vi "LOGIC_CheckStopCond.vi"(8 "error in (no error)":errorcluster, 11 "Database RefNum in":T1) -> (0 "error out":errorcluster)   [LabVIEW 2016]
uses:
  DBSHAND/private/vis/DatabaseHand_RefNum.ctl
  DBSHAND/private/vis/DatabaseHand_Element_Get(bool).vi
  DBSHAND/private/vis/DatabaseHand_Element_Set(I32).vi
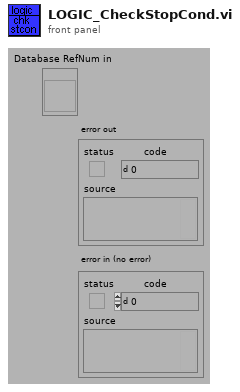
[diagram p1: front panel]
types:
  T1 = typedef "DatabaseHand_RefNum.ctl" = refnum<vi>
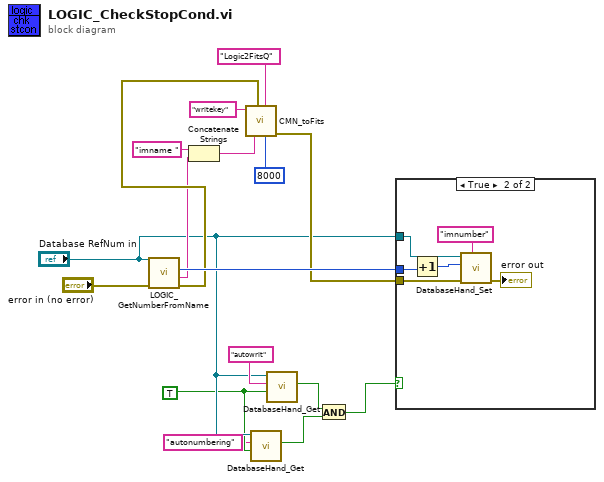
[diagram p0: block diagram]
diagram:
  w4 = TRUE
  n1 = call "LOGIC_GetNumberFromName.vi"("error in (no error)"="error in (no error)", "Database RefNum in"="Database RefNum in") -> ("error out"=w12:errorcluster, "lastimg"=w8:string, "number"=w13:i32)  [unwired: 7 out]
  n2 = Concatenate Strings("imname " ("string"), w8) -> (w15:string)
  n3 = call "CMN_toFits.vi"("ms timeout (-1)"=8000, "response Q"="Logic2FitsQ", "key"=w15, "error in (no error)"=w12, "command"="writekey") -> ("error out"=w11:errorcluster)  [unwired: 3 in, 3 out]
  n4 = call-poly "DatabaseHand_Get.vi"("default value"=w4, "name"="autonumbering", "Database RefNum in"="Database RefNum in") -> ("value"=w2:bool)  [unwired: 2 in, 6 out]
  n5 = call-poly "DatabaseHand_Get.vi"("default value"=w4, "name"="autowrit", "Database RefNum in"="Database RefNum in") -> ("value"=w6:bool)  [unwired: 2 in, 6 out]
  n6 = And(x=w6, y=w2) -> (x .and. y?=w1:bool)
  n7 = case shown="True" w1 {
    tunnel: w13 -> [_ w20]
    tunnel: w11 -> [_ w19]
    tunnel: "Database RefNum in" -> [_ w18]
    frame False {
    }
    frame True {
      n8 = Increment(x=w20) -> (x+1=w22:i32)
      n9 = call-poly "DatabaseHand_Set.vi"("name"="imnumber", "error in (no error)"=w19, "value"=w22, "Database RefNum in"=w18) -> ("error out"=→"error out":errorcluster)  [unwired: 4 in, 3 out]
    }
  }
